vi "Close.vi"(8 "error in (no error)":errorcluster, 11 "Data in":refnum<class "DAQmx-Bus.lvclass">) -> (0 "error out":errorcluster, 3 "Data out":refnum<class "DAQmx-Bus.lvclass">)   [LabVIEW 2021, in "DAQmx-Bus.lvclass"]
doc: "Abstract Data Classes 2.1.1.13\nTim Streeter - TSA\nCopyright (c) 2025, TSA"
uses:
  DAQmx-Bus.lvclass
  DAQmx-Bus.lvclass/DAQmx-Bus.ctl
  Properties/Read Stop.vi
  Properties/Read Sync.vi
  Properties/Read Actor Ref.vi
  Properties/Write Actor Ref.vi
  <vilib>/TSA/Omni-Bus/Omni-Bus/Bus Access/Bus_Access.lvclass
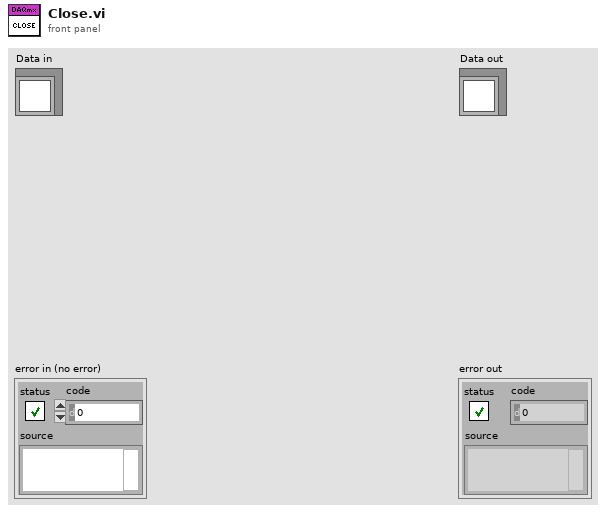
[diagram p1: front panel]
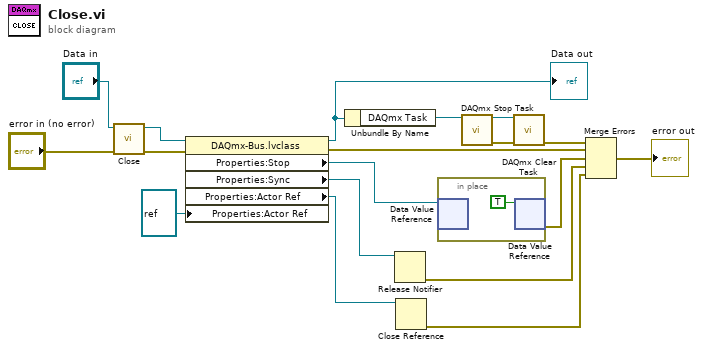
[diagram p0: block diagram]
diagram:
  n1 = call-parent "Close.vi"("error in (no error)"="error in (no error)", "Data in"="Data in") -> ("error out"=w16:errorcluster, "Data out"=w15:refnum<class "DAQmx-Bus.lvclass">)  [unwired: 8 in]
  n2 = property class="DAQmx-Bus.lvclass"(reference=w15, error in=w16, "Properties:Actor Ref"=refnum<vi> refnum ("Actor Ref")) -> (reference out=w5:refnum<class "DAQmx-Bus.lvclass">, error out=w10:errorcluster, "Properties:Stop"=w13:refnum<data-value>, "Properties:Sync"=w12:refnum<notifier>, "Properties:Actor Ref"=w11:refnum<vi>)
  "Data out" <- w5
  n3 = Unbundle By Name(w5) -> ("DAQmx Task"=w1:refnum<k21>)
  n4 = Release Notifier(notifier=w12) -> (error out=w8:errorcluster)  [unwired: 2 in, 2 out]
  n5 = Close Reference(reference=w11) -> (error out=w7:errorcluster)  [unwired: 1 in]
  n6 = in-place {
    n7 = in-place-dvr #1(w13) -> ()  [unwired: 2 out]
    n8 = in-place-dvr #1(TRUE ("data value")) -> (w9:errorcluster)  [unwired: 1 out]
  }
  n9 = call <vilib>:"DAQmx Stop Task.vi"("task/channels in"=w1) -> ("task out"=w3:refnum<k21>, "error out"=w2:errorcluster)  [unwired: 13 in]
  n10 = call <vilib>:"DAQmx Clear Task.vi"("task in"=w3, "error in"=w2) -> ("error out"=w4:errorcluster)  [unwired: 13 in]
  n11 = Merge Errors(w4, w10, w9, w8, w7) -> (→"error out":errorcluster)
